vi "get emf settings.vi"(8 "error in (no error)":errorcluster, 10 "emf_settings":T1, 11 "id":i32) -> (0 "error out":errorcluster, 2 "emf_settings out":T1, 3 "function return":i32)   [LabVIEW 2012, in "libximc.lvlib"]
doc: "result_t XIMC_API get_emf_settings (device_t id, emf_settings_t* emf_settings);"
uses:
  libximc.lvlib
  libximc.dll
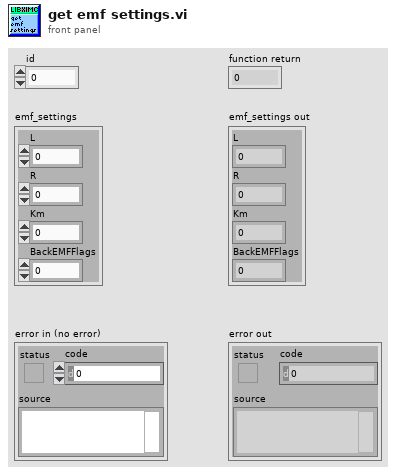
[diagram p1: front panel]
types:
  T1 = cluster{"L":sgl, "R":sgl, "Km":sgl, "BackEMFFlags":u32}
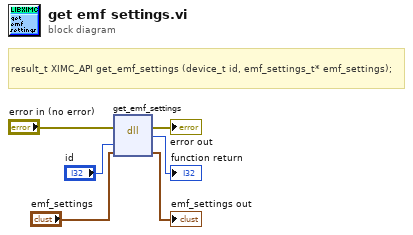
[diagram p0: block diagram]
diagram:
  # "result_t XIMC_API get_emf_settings (device_t id, emf_settings_t* emf_settings);"
  n1 = dll-call lib="E:/labview-2.12.1-Labview_12.0/ximcLVx32/libximc.*" fn="get_emf_settings"(error in="error in (no error)", "id"="id", "emf_settings"="emf_settings") -> (error out=→"error out":errorcluster, →"function return":i32, "emf_settings"=→"emf_settings out":T1)  [unwired: 3 in, 1 out]
